vi "Sub 1.vi"(8 "error in (no error)":errorcluster, 11 "data value reference":refnum<data-value>) -> (0 "error out":errorcluster, 3 "data value reference out":refnum<data-value>)   [LabVIEW 2009]
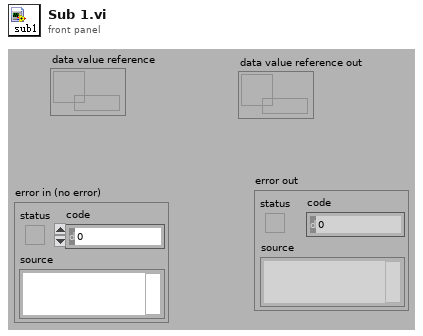
[diagram p1: front panel]
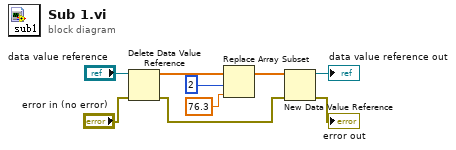
[diagram p0: block diagram]
diagram:
  n1 = Delete Data Value Reference(data value reference="data value reference", error in="error in (no error)") -> (data value=w8:dbl[], error out=w3:errorcluster)
  n2 = Replace Array Subset(array=w8, new element=76.3 ("new element/subarray"), index=2) -> (w5:dbl[])
  n3 = New Data Value Reference(data value=w5, error in=w3) -> (data value reference=→"data value reference out":refnum<data-value>, error out=→"error out":errorcluster)
